vi "S2C_ExeScriptPause.vi"(8 "Error In":errorcluster, 11 "Q-Ref":refnum<queue>) -> (0 "Error Out":errorcluster)   [LabVIEW 2015]
doc: "Pauses the executable script execution."
uses:
  Controls/S2C_ResultStatus.ctl
  Controls/S2C_ExePause.ctl
  Globals/S2C_Globals.vi
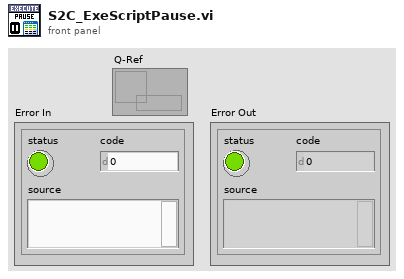
[diagram p1: front panel]
types:
  T1 = typedef "S2C_ExePause.ctl" = bool
  T2 = typedef "S2C_ResultStatus.ctl" = enum16{"Passed", "Failed", "Logged", "Aborted", "Error", "Testing...", "Paused", "No Record"}
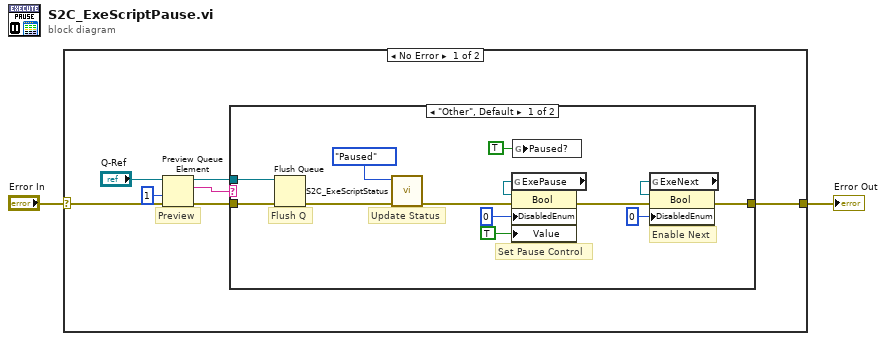
[diagram p0: block diagram]
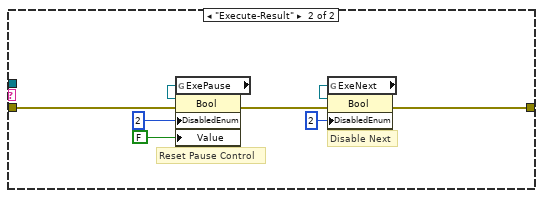
[diagram p2: hidden frame]
diagram:
  n1 = case shown="No Error" "Error In" {
    selector: "Error In" -> [w9 w31]
    tunnel: [w4 w31] -> w1
    frame No Error {
      # "Preview"
      n2 = Preview Queue Element(queue="Q-Ref", timeout in ms (-1)=1, error in (no error)=w9) -> (queue out=w6:refnum<queue>, element=w5:string, error out=w7:errorcluster)  [unwired: 1 out]
      n3 = case shown="\"Other\", Default" w5 {
        tunnel: [w16 w23] -> w4
        tunnel: w7 -> [w22 w26]
        tunnel: w6 -> [w21 _]
        frame "Other", Default {
          # "Set Pause Control"
          # "Update Status"
          # "Enable Next"
          # "Flush Q"
          n4 = Flush Queue(queue=w21, error in (no error)=w22) -> (error out=w17:errorcluster)  [unwired: 2 out]
          n5 = call "S2C_ExeScriptStatus.vi"("Error In"=w17, "Status"=S2C_ResultStatus."Paused") -> ("Error Out"=w14:errorcluster)  [unwired: 9 in]
          n6 = global read "S2C_Globals.vi" "ExePause"() -> (w15:refnum<vi>)
          n7 = property on="Property Node" class="Bool"(reference=w15, error in=w14, "DisabledEnum"=u8 0, "Value"=T1 TRUE) -> (error out=w13:errorcluster)  [unwired: 1 out]
          n8 = global write "S2C_Globals.vi" "Paused?"(TRUE ("Paused?")) -> ()
          n9 = global read "S2C_Globals.vi" "ExeNext"() -> (w20:refnum<vi>)
          n10 = property on="Property Node" class="Bool"(reference=w20, error in=w13, "DisabledEnum"=u8 0) -> (error out=w16:errorcluster)  [unwired: 1 out]
        }
        frame "Execute-Result" {
          # "Reset Pause Control"
          # "Disable Next"
          n11 = global read "S2C_Globals.vi" "ExePause"() -> (w27:refnum<vi>)
          n12 = property on="Property Node" class="Bool"(reference=w27, error in=w26, "DisabledEnum"=u8 2, "Value"=T1 FALSE) -> (error out=w24:errorcluster)  [unwired: 1 out]
          n13 = global read "S2C_Globals.vi" "ExeNext"() -> (w30:refnum<vi>)
          n14 = property on="Property Node" class="Bool"(reference=w30, error in=w24, "DisabledEnum"=u8 2) -> (error out=w23:errorcluster)  [unwired: 1 out]
        }
      }
    }
    frame Error {
    }
  }
  "Error Out" <- w1
